vi "Conf-Sensor.vi"(7 "Slave Address (7-bit)":u8, 8 "error in (no error)":errorcluster, 11 "I2C Ref Out in":T1) -> (0 "error out":errorcluster, 3 "I2C Ref Out out":T1, 4 "ChipID":u8[](array[numeric]) format="%x")   [LabVIEW 2015]
uses:
  <vilib>/myRIO/Instrument Drivers/Onboard IO/I2C/typedefs/I2C Reference.ctl
  <vilib>/myRIO/Common/Instrument Driver Framework/Utilities/typedefs/myRIO Generic Hardware Reference.ctl
  <vilib>/myRIO/Common/Instrument Driver Framework/Utilities/typedefs/Hardware Version Enum.ctl
  <vilib>/myRIO/Common/Instrument Driver Framework/Utilities/typedefs/myRIO v1.0 Reference.ctl
  <vilib>/myRIO/Common/Instrument Driver Framework/Utilities/typedefs/Generic FPGA Reference.ctl
  <vilib>/myRIO/Common/Instrument Driver Framework/myRIO v1.0/I2C/typedefs/I2C Channels Enum.ctl
  <vilib>/myRIO/Instrument Drivers/Onboard IO/I2C/typedefs/I2C Configuration.ctl
  <vilib>/myRIO/Instrument Drivers/Onboard IO/I2C/typedefs/I2C Transfer Rate.ctl
  <vilib>/Utility/error.llb/Error Cluster From Error Code.vi
  <vilib>/myRIO/Common/Instrument Driver Framework/myRIO v1.0/I2C/vis/myRIO v1.0 Write I2C.vi
  <vilib>/myRIO/Common/Instrument Driver Framework/myRIO v1.0/I2C/vis/myRIO v1.0 Read I2C.vi
  <vilib>/myRIO/Instrument Drivers/Onboard IO/I2C/I2C.lvlib
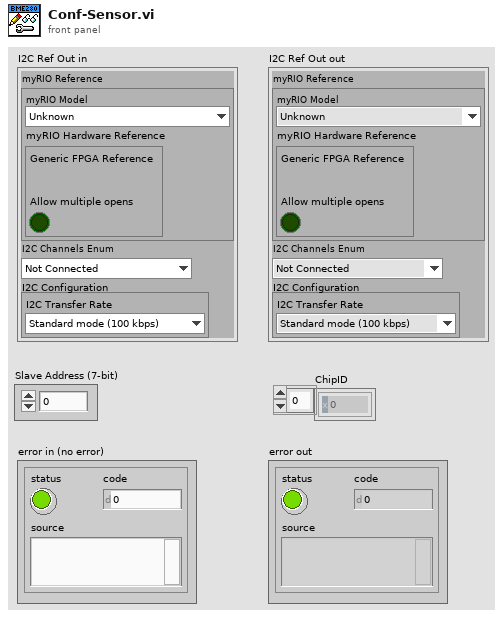
[diagram p1: front panel]
types:
  T1 = typedef "I2C.lvlib/I2C Reference.ctl" = cluster{"myRIO Reference":T2, "I2C Channels Enum":T6, "I2C Configuration":T7}
  T2 = typedef "myRIO Generic Hardware Reference.ctl" = cluster{"myRIO Model":T3, "myRIO Hardware Reference":T4}
  T3 = typedef "Hardware Version Enum.ctl" = enum16{"Unknown", "myRIO-1900", "myRIO-1950", "roboRIO"}
  T4 = typedef "myRIO v1.0 Reference.ctl" = cluster{"Generic FPGA Reference":T5, "Allow multiple opens":bool}
  T5 = typedef "Generic FPGA Reference.ctl" = refnum<k20>
  T6 = typedef "I2C Channels Enum.ctl" = enum16{"Not Connected", "A/I2C", "B/I2C", "I2C/I2C"}
  T7 = typedef "I2C.lvlib/I2C Configuration.ctl" = cluster{"I2C Transfer Rate":T8}
  T8 = typedef "I2C.lvlib/I2C Transfer Rate.ctl" = enum16{"Standard mode (100 kbps)", "Fast mode (400 kbps)"}
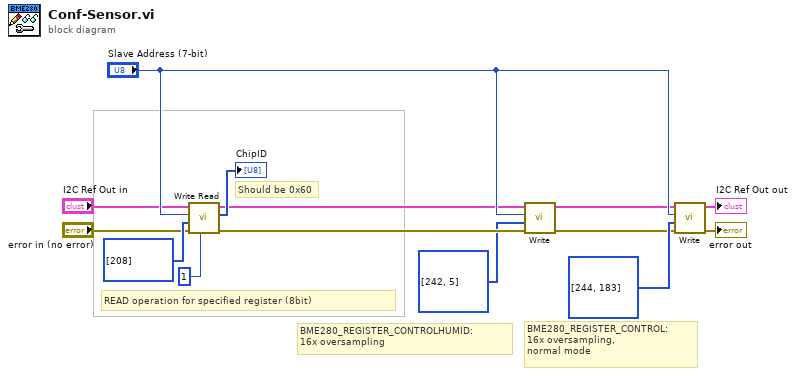
[diagram p0: block diagram]
diagram:
  # "READ operation for specified register (8bit)"
  # "BME280_REGISTER_CONTROL:\n16x oversampling,\nnormal mode"
  # "BME280_REGISTER_CONTROLHUMID:\n16x oversampling"
  # "Should be 0x60"
  n1 = call <vilib>:"Write Read.vi"("Byte Count"=u32 1, "error in (no error)"="error in (no error)", "Bytes to Write"=u8[] [208], "Slave Address (7-bit)"="Slave Address (7-bit)", "I2C Ref In"="I2C Ref Out in") -> ("error out"=w10:errorcluster, "Bytes Read"=→"ChipID":u8[], "I2C Ref Out"=w8:T1)  [unwired: 3 in]
  n2 = call <vilib>:"Write.vi"("error in (no error)"=w10, "Bytes to Write"=u8[] [242, 5], "Slave Address (7-bit)"="Slave Address (7-bit)", "I2C Ref In"=w8) -> ("error out"=w2:errorcluster, "I2C Ref Out"=w1:T1)  [unwired: 6 in]
  n3 = call <vilib>:"Write.vi"("error in (no error)"=w2, "Bytes to Write"=u8[] [244, 183], "Slave Address (7-bit)"="Slave Address (7-bit)", "I2C Ref In"=w1) -> ("error out"=→"error out":errorcluster, "I2C Ref Out"=→"I2C Ref Out out":T1)  [unwired: 6 in]
